vi "Get Next Unique Item Label.vi"(8 "error in (no error)":errorcluster, 9 "Start Value (1)":i32=1, 10 "Label":string, 11 "Parent Ref in":T1=18446744073709551615 format="%.0x") -> (0 "error out":errorcluster, 2 "Label out":string, 3 "Parent Ref dup":T1=18446744073709551615 format="%.0x", 4 "Next value":i32)   [LabVIEW 2017, in "PXImc System Explorer.lvlib"]
uses:
  PXImc System Explorer.lvlib
  <vilib>/NI Veristand/Custom Device API/Custom Device Item Ref.ctl
  <vilib>/NI VeriStand/Custom Device API/Custom Device API.lvlib
panel:
  in  "format string":string=" %d"
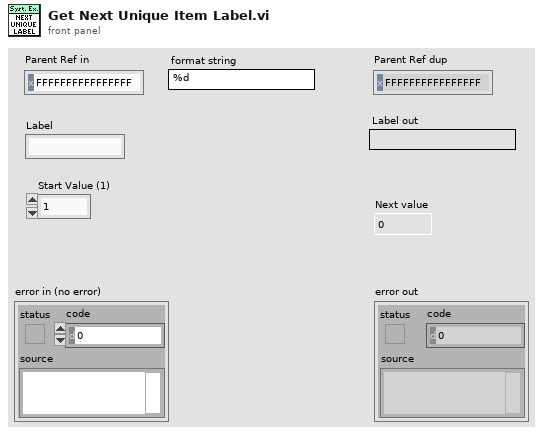
[diagram p1: front panel]
types:
  T1 = typedef "Custom Device API.lvlib/Custom Device Item Ref.ctl" = u64
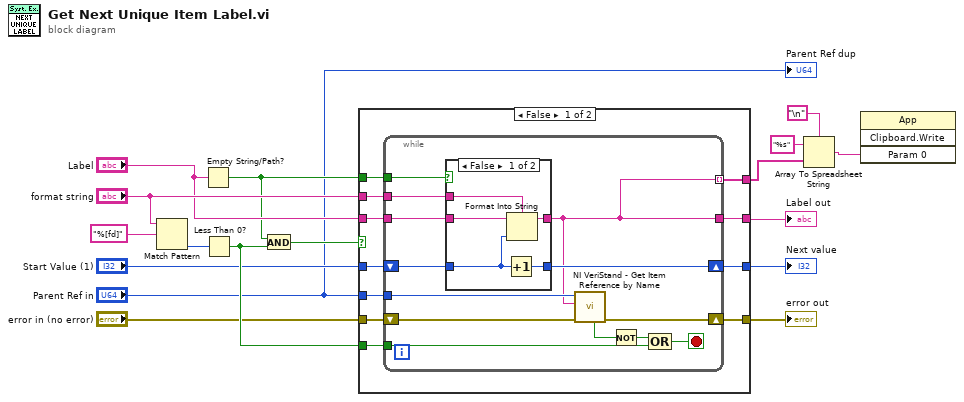
[diagram p0: block diagram]
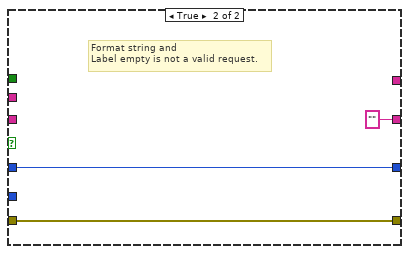
[diagram p3: hidden frame]
diagram:
  n1 = Match Pattern(string="format string", regular expression="%[fd]") -> (offset past match=w14:i32)  [unwired: 1 in, 3 out]
  n2 = Empty String/Path?(string/path="Label") -> (empty?=w10:bool)
  n3 = Less Than 0?(x=w14) -> (x < 0?=w11:bool)
  n4 = And(x=w10, y=w11) -> (x .and. y?=w9:bool)
  n5 = case shown="False" w9 {
    tunnel: "Parent Ref in" -> [w28 _]
    tunnel: [w27 "" ("Label")] -> w17
    tunnel: "Start Value (1)" -> [w26 w50]
    tunnel: "format string" -> [w25 _]
    tunnel: w11 -> [w24 _]
    tunnel: "Label" -> [w23 _]
    tunnel: w10 -> [w22 _]
    tunnel: [w21 w50] -> w12
    tunnel: "error in (no error)" -> [w20 w49]
    tunnel: [w19 w49] -> w6
    tunnel: [w18 _] -> w4
    frame False {
      n6 = while {
        shift-right: [w33] -> w21
        shift-left: w26 -> [w41]
        tunnel: w23 -> [w40]
        tunnel: w28 -> [w32]
        tunnel: [w29] -> w27
        tunnel: w25 -> [w39]
        tunnel: w24 -> [w35]
        tunnel: w22 -> [w34]
        shift-right: [w30] -> w19
        shift-left: w20 -> [w31]
        tunnel: [w29] -> w18 mode=indexing
        stop <- w36 stop-if-true
        n7 = case shown="False" w34 {
          tunnel: w41 -> [w43 w47]
          tunnel: [w46 w48] -> w29
          tunnel: w40 -> [w45 w48]
          tunnel: w39 -> [w44 _]
          tunnel: [w42 w47] -> w33
          frame False {
            n8 = Increment(x=w43) -> (x+1=w42:i32)
            n9 = Format Into String(format string=w44, initial string=w45, w43) -> (resulting string=w46:string)  [unwired: 1 in, 1 out]
          }
          frame True {
          }
        }
        n10 = call <vilib>:"NI VeriStand - Get Item Reference by Name.vi"("error in (no error)"=w31, "Item Name"=w29, "Parent Ref in"=w32) -> ("error out"=w30:errorcluster, "Found"=w38:bool)  [unwired: 5 in, 2 out]
        n11 = Not(x=w38) -> (.not. x?=w37:bool)
        n12 = Compound Arithmetic op=OR(w37, w35) -> (w36:bool)
      }
    }
    frame True {
      # "Format string and\nLabel empty is not a valid request."
    }
  }
  "Label out" <- w17
  "error out" <- w6
  "Next value" <- w12
  n13 = Array To Spreadsheet String(delimiter (Tab)="\n", array=w4, 3:"%s" ("format string")) -> (spreadsheet string=w1:string)
  n14 = invoke class="App" method="Clipboard.Write"("Param 0"=w1) -> ()  [unwired: 3 in, 4 out]
  "Parent Ref dup" <- "Parent Ref in"
